vi "Search Ordered Table.vi"(9 "starting index":i32, 10 "x value":dbl, 11 "ordered x array":dbl[](array[numeric]) format="%_6g") -> (3 "fractional index":dbl format="%_6g")   [LabVIEW 2013, in "NI_Gmath.lvlib"]
doc: "Works on the assumption that <B>ordered x array</B> is in monotonically increasing or decreasing order and can therefore efficiently search for the relative index of the location of <B>x value</B> within the <B>x array</B>. The VI starts the search at the <B>starting index</B> and begins by using a fast hunting phase to roughly bracket the location and then narrows to the final bracket using a bisection search. The VI computes the <B>fractional index</B> location by using linear interpolation."
uses:
  NI_Gmath.lvlib
panel:
  # "Search Ordered Table"
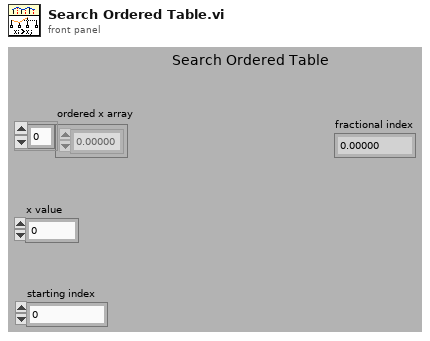
[diagram p1: front panel]
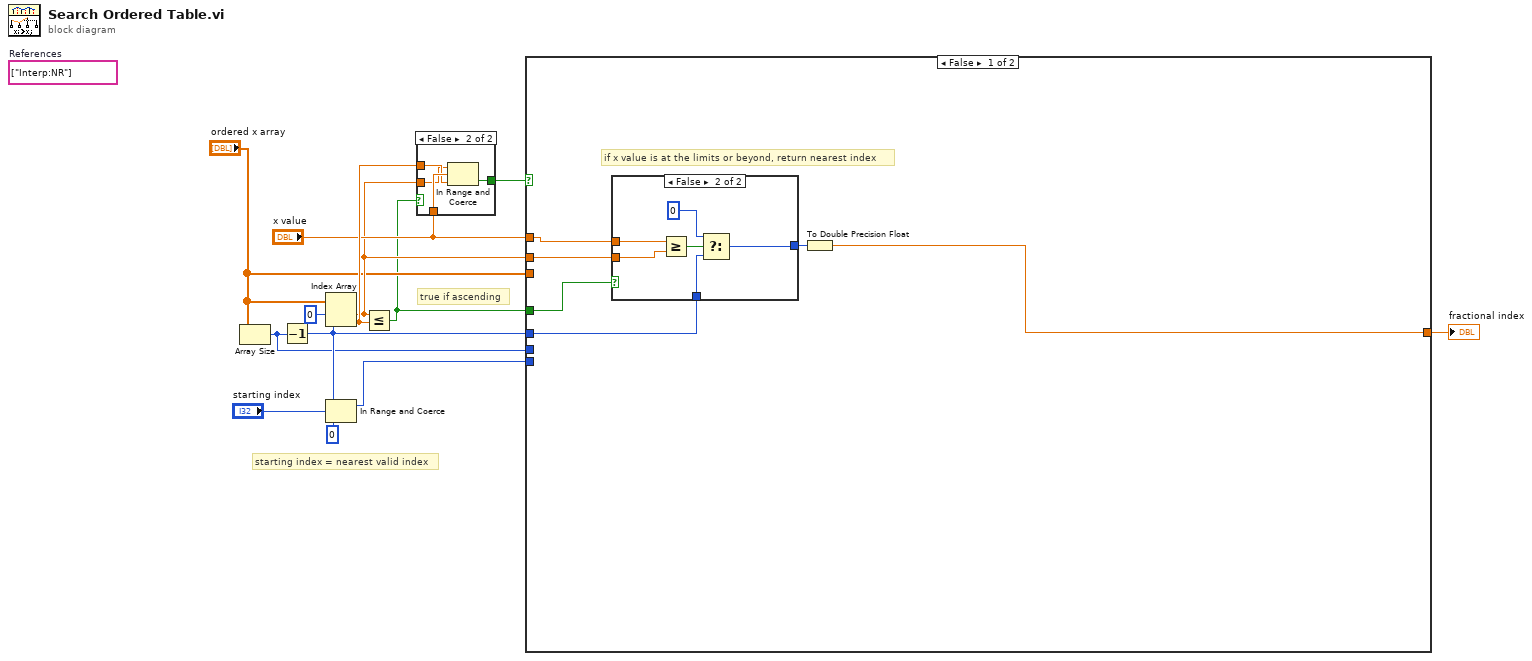
[diagram p0: block diagram]
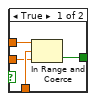
[diagram p2: hidden frame]
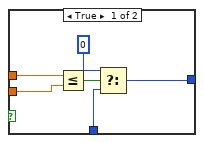
[diagram p3: hidden frame]
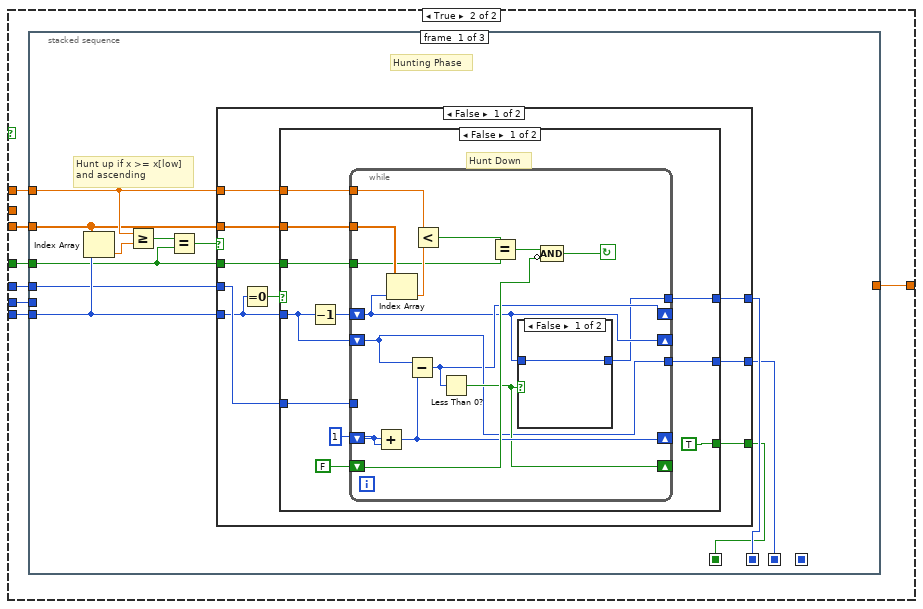
[diagram p4: hidden frame]
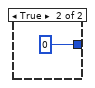
[diagram p5: hidden frame]
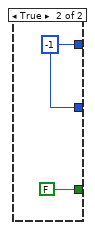
[diagram p6: hidden frame]
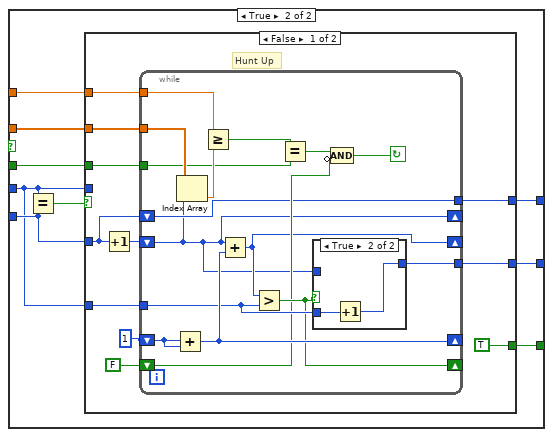
[diagram p7: hidden frame]
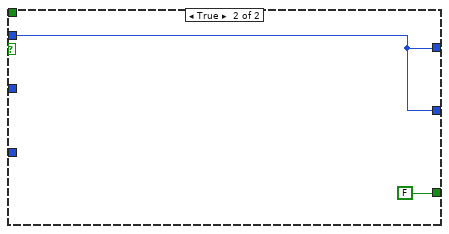
[diagram p9: hidden frame]
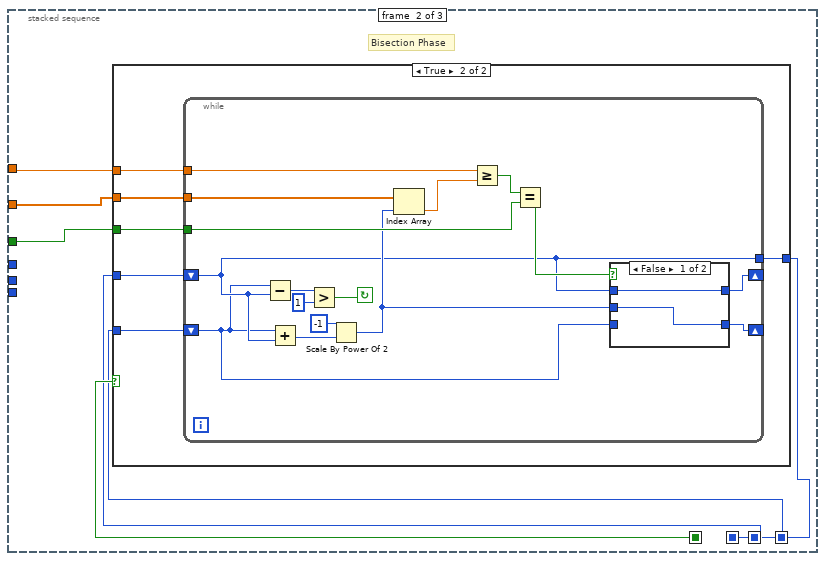
[diagram p10: hidden frame]
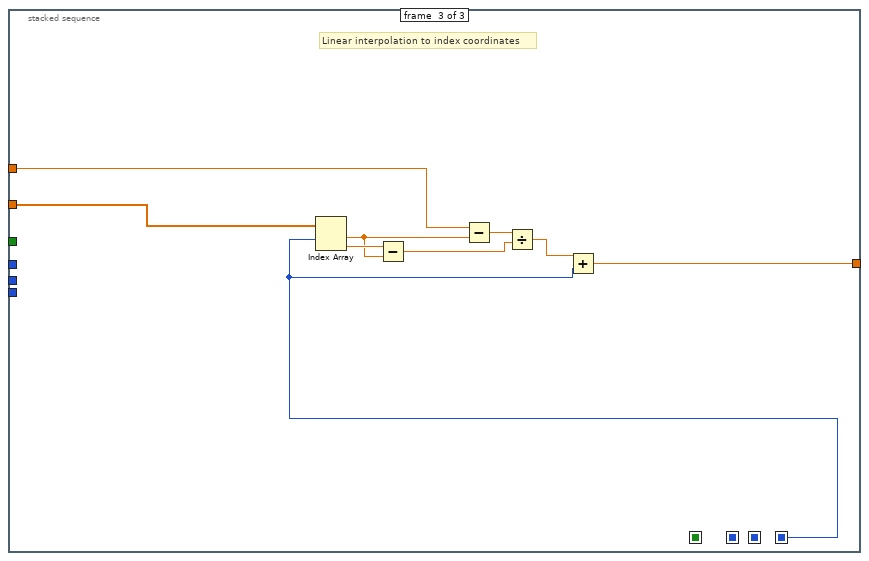
[diagram p13: hidden frame]
diagram:
  (unwired) string[] ["Interp:NR"]  # References
  # "starting index = nearest valid index"
  # "true if ascending"
  n1 = Array Size(array="ordered x array") -> (size(s)=w10:i32)
  n2 = Decrement(x=w10) -> (x-1=w11:i32)
  n3 = Index Array(array="ordered x array", index #1=0 ("index"), index #2=w11) -> (element #1=w6:dbl, element #2=w9:dbl)
  n4 = In Range and Coerce(upper limit=w11, x="starting index", lower limit=0 ("index")) -> (coerced(x)=w3:i32)  [unwired: 1 out]
  n5 = Less Or Equal?(x=w6, y=w9) -> (x <= y?=w1:bool)
  n6 = case shown="False" w1 {
    tunnel: w9 -> [w17 w19]
    tunnel: "x value" -> [w16 w21]
    tunnel: [w15 w20] -> w7
    tunnel: w6 -> [w14 w18]
    frame True {
      n7 = In Range and Coerce(upper limit=w17, x=w16, lower limit=w14) -> (In Range?=w15:bool)  [unwired: 1 out]
    }
    frame False {
      n8 = In Range and Coerce(upper limit=w18, x=w21, lower limit=w19) -> (In Range?=w20:bool)  [unwired: 1 out]
    }
  }
  n9 = case shown="False" w7 {
    tunnel: "x value" -> [w27 w46]
    tunnel: "ordered x array" -> [_ w45]
    tunnel: w3 -> [_ w44]
    tunnel: w1 -> [w23 w43]
    tunnel: w11 -> [w25 w42]
    tunnel: w10 -> [_ w41]
    tunnel: w6 -> [w26 _]
    tunnel: [w22 w40] -> w5
    frame False {
      # "if x value is at the limits or beyond, return nearest index"
      n10 = case shown="False" w23 {
        tunnel: w27 -> [w33 w39]
        tunnel: w26 -> [w32 w38]
        tunnel: w25 -> [w29 w34]
        tunnel: [w28 w36] -> w24
        frame True {
          n11 = Less Or Equal?(x=w33, y=w32) -> (x <= y?=w31:bool)
          n12 = Select(t=0 ("index"), s=w31, f=w29) -> (s? t:f=w28:i32)
        }
        frame False {
          n13 = Greater Or Equal?(x=w39, y=w38) -> (x >= y?=w37:bool)
          n14 = Select(t=0 ("index"), s=w37, f=w34) -> (s? t:f=w36:i32)
        }
      }
      n15 = To Double Precision Float(number=w24) -> (double precision float=w22:dbl)
    }
    frame True {
      n16 = stacked-sequence {
        seq-local: [w52 _ _] -> [_ w143 _]
        seq-local: [w51 _ _] -> [_ w142 _]
        seq-local: [w50 _ _] -> [_ w144 _]
        seq-local: [_ w138 _] -> [_ _ w173]
        tunnel: w46 -> [w57 w140 w178]
        tunnel: w45 -> [w56 w141 w180]
        tunnel: w44 -> [w55 _ _]
        tunnel: w43 -> [w54 w139 _]
        tunnel: w42 -> [w53 _ _]
        tunnel: w41 -> [_ _ _]
        tunnel: [_ _ w172] -> w40
        frame #0 {
          # "Hunt up if x >= x[low]\nand ascending"
          # "Hunting Phase"
          n17 = Index Array(array=w56, index=w55) -> (element=w49:dbl)
          n18 = Greater Or Equal?(x=w57, y=w49) -> (x >= y?=w48:bool)
          n19 = Equal?(x=w48, y=w54) -> (x = y?=w47:bool)
          n20 = case shown="False" w47 {
            tunnel: w53 -> [w61 w98]
            tunnel: w55 -> [w60 w105]
            tunnel: w57 -> [w66 w104]
            tunnel: w56 -> [w65 w103]
            tunnel: w54 -> [w64 w102]
            tunnel: [w63 w101] -> w52
            tunnel: [w62 w100] -> w51
            tunnel: [w58 w97] -> w50
            frame False {
              n21 = Equal To 0?(x=w60) -> (x = 0?=w59:bool)
              n22 = case shown="False" w59 {
                tunnel: w66 -> [w77 _]
                tunnel: w65 -> [w76 _]
                tunnel: w64 -> [w75 _]
                tunnel: [w72 w96] -> w63
                tunnel: [w71 w96] -> w62
                tunnel: w61 -> [w69 _]
                tunnel: w60 -> [w68 _]
                tunnel: [TRUE FALSE] -> w58
                frame False {
                  # "Hunt Down"
                  n23 = Decrement(x=w68) -> (x-1=w73:i32)
                  n24 = while {
                    shift-right: [w83] -> _
                    shift-left: 1 ("index") -> [w87]
                    shift-right: [w80] -> _
                    shift-left: w73 -> [w79]
                    shift-right: [w79] -> _
                    shift-left: w68 -> [w81]
                    tunnel: w77 -> [w91]
                    tunnel: w76 -> [w92]
                    tunnel: w75 -> [w89]
                    tunnel: w69 -> [_]
                    tunnel: [w78] -> w72
                    tunnel: [w81] -> w71
                    shift-right: [w82] -> _
                    shift-left: FALSE -> [w84]
                    stop <- w85 continue-if-true
                    n25 = Add(x=w87, y=w87) -> (x+y=w83:i32)
                    n26 = Index Array(array=w92, index=w79) -> (element=w90:dbl)
                    n27 = Subtract(x=w81, y=w83) -> (x-y=w80:i32)
                    n28 = Less?(x=w91, y=w90) -> (x < y?=w88:bool)
                    n29 = Less Than 0?(x=w80) -> (x < 0?=w82:bool)
                    n30 = Equal?(x=w88, y=w89) -> (x = y?=w86:bool)
                    n31 = case shown="False" w82 {
                      tunnel: [w93 0] -> w78
                      tunnel: w79 -> [w93 _]
                      frame False {
                      }
                      frame True {
                      }
                    }
                    n32 = Compound Arithmetic op=AND(w86, invert w84) -> (w85:bool)
                  }
                }
                frame True {
                  w96 = -1
                }
              }
            }
            frame True {
              n33 = Equal?(x=w98, y=w105) -> (x = y?=w99:bool)
              n34 = case shown="False" w99 {
                tunnel: w105 -> [w115 _]
                tunnel: w104 -> [w114 _]
                tunnel: w103 -> [w113 _]
                tunnel: w102 -> [w112 _]
                tunnel: w98 -> [w110 _]
                tunnel: [w109 w137] -> w101
                tunnel: [w108 w137] -> w100
                tunnel: w98 -> [_ w137]
                tunnel: [TRUE FALSE] -> w97
                frame False {
                  # "Hunt Up"
                  n35 = Increment(x=w115) -> (x+1=w116:i32)
                  n36 = while {
                    shift-right: [w125] -> _
                    shift-left: 1 ("index") -> [w127]
                    shift-right: [w118] -> _
                    shift-left: w115 -> [w120]
                    shift-right: [w119] -> _
                    shift-left: w116 -> [w118]
                    tunnel: w114 -> [w131]
                    tunnel: w113 -> [w132]
                    tunnel: w112 -> [w129]
                    tunnel: w110 -> [w124]
                    tunnel: [w120] -> w109
                    tunnel: [w117] -> w108
                    shift-right: [w122] -> _
                    shift-left: FALSE -> [w121]
                    stop <- w123 continue-if-true
                    n37 = Add(x=w127, y=w127) -> (x+y=w125:i32)
                    n38 = Index Array(array=w132, index=w118) -> (element=w130:dbl)
                    n39 = Greater Or Equal?(x=w131, y=w130) -> (x >= y?=w128:bool)
                    n40 = Add(x=w118, y=w125) -> (x+y=w119:i32)
                    n41 = Greater?(x=w119, y=w124) -> (0:w122:bool)
                    n42 = Equal?(x=w128, y=w129) -> (x = y?=w126:bool)
                    n43 = case shown="True" w122 {
                      tunnel: w124 -> [_ w135]
                      tunnel: w118 -> [w133 _]
                      tunnel: [w133 w134] -> w117
                      frame False {
                      }
                      frame True {
                        n44 = Increment(x=w135) -> (x+1=w134:i32)
                      }
                    }
                    n45 = Compound Arithmetic op=AND(w126, invert w121) -> (w123:bool)
                  }
                }
                frame True {
                }
              }
            }
          }
        }
        frame #1 {
          # "Bisection Phase"
          n46 = case shown="True" w144 {
            tunnel: w143 -> [w145 w151]
            tunnel: w142 -> [_ w150]
            tunnel: [w145 w149] -> w138
            tunnel: w141 -> [_ w148]
            tunnel: w140 -> [_ w147]
            tunnel: w139 -> [_ w146]
            frame False {
            }
            frame True {
              n47 = while {
                shift-right: [w155] -> _
                shift-left: w151 -> [w153]
                shift-right: [w154] -> _
                shift-left: w150 -> [w152]
                tunnel: [w153] -> w149
                tunnel: w148 -> [w162]
                tunnel: w147 -> [w161]
                tunnel: w146 -> [w159]
                stop <- w165 continue-if-true
                n48 = Subtract(x=w152, y=w153) -> (x-y=w167:i32)
                n49 = Add(x=w152, y=w153) -> (x+y=w164:i32)
                n50 = Greater?(x=w167, y=1) -> (0:w165:bool)
                n51 = Scale By Power Of 2(n=-1, x=w164) -> (x*2^n=w156:i32)
                n52 = Index Array(array=w162, index=w156) -> (element=w160:dbl)
                n53 = Greater Or Equal?(x=w161, y=w160) -> (x >= y?=w158:bool)
                n54 = Equal?(x=w158, y=w159) -> (x = y?=w157:bool)
                n55 = case shown="False" w157 {
                  tunnel: w156 -> [w169 w171]
                  tunnel: [w168 w171] -> w155
                  tunnel: [w169 w170] -> w154
                  tunnel: w152 -> [_ w170]
                  tunnel: w153 -> [w168 _]
                  frame False {
                  }
                  frame True {
                  }
                }
              }
            }
          }
        }
        frame #2 {
          # "Linear interpolation to index coordinates"
          n56 = Index Array(array=w180, index #1=w173) -> (element #1=w177:dbl, element #2=w179:dbl)  [unwired: 1 in]
          n57 = Subtract(x=w179, y=w177) -> (x-y=w175:dbl)
          n58 = Subtract(x=w178, y=w177) -> (x-y=w176:dbl)
          n59 = Divide(x=w176, y=w175) -> (x/y=w174:dbl)
          n60 = Add(x=w174, y=w173) -> (x+y=w172:dbl)
        }
      }
    }
  }
  "fractional index" <- w5
